vi "Open_File_for_write_check.vi"(8 "advisory dialog? (display:T)":bool=TRUE, 9 "append to file? (new file:F)":bool, 11 "file path":path) -> (0 "error out":errorcluster, 3 "refnum":refnum<file>)   [LabVIEW 2015]
doc: "Opens an existing file, creates a new file, or replaces an existing file, programmatically or interactively using dialog. You can optionally specify a dialog prompt, default file name, start path, or filter pattern, and you can specify open and deny modes when opening a file, plus group and permission when creating a new file. Use this VI with the intermediate Write File+ or Read File+ VIs described below.\n\nfile path is the path name of the file. If file path is empty (default value) or is Not A Path, the VI displays a File dialog box from which you can select a file. Error 43 occurs if the user cancels the dialog. \n\nfunction is the operation to perform:\n\n 0 (open) opens an existing file. Error 7 occurs if the file cannot be found.\n \n 1 (open or create) opens an existing file or creates a new file if one does not exist.\n\n 2 (create or replace) creates a new file or replaces a file if it exists and you give permission. Replacement is done by opening the file and setting EOF to 0. Error 43 occurs if the user elects to disallow the replacement using dialog. \n\n 3 (create) creates a new file. Error 8 occurs if the file already exists.\n\nadvisory dialog? Set TRUE (default) if you want a dialog if function=0 and the file does not exist, or if function=2 or 3 and the file exists.\n\nprompt is the message that appears below the list of files and directories in the file dialog.\n\ndefault name is the initial file name that appears in the selection box of the file dialog.\n\nstart path is the path name to the initially displayed directory in a file dialog. The default value is Not A Path, which is the path to the last directory shown in a file dialog.\n\npattern is the match pattern specification to display only certain types of files or directories. See the description of the File Dialog function for more information.\n\nerror in is a cluster of three elements (error?, code, and source) that describe the upstream error state, that is, the existance of any error preceeding the execution of the VI. The VI executes normally only if no incoming error exists; otherwise it merely passes the error in value to error out. error? is TRUE if an error occurred; the default value is FALSE. code is the error code; the default value is 0. source is in most cases the name of the VI or function that produced the error; the default value is an empty string.\n\nnew file path is the path of the file opened or created. You can use this output to determine the path of a file that you open or create using dialog. new file path returns Not A Path if the user selects Cancel from the dialog box.\n\nrefnum is the reference number of the open file. The value is Not A Refnum if the file cannot be opened.\n\nfile size is the size of the file in bytes; it is also the location of the end of file.\n\nerror out is a cluster of three elements (error?, code, and source) that describe the error state following the execution of the VI. If an incoming error does not exist, the VI executes normally and error out describes the VI's error state; if an incoming error exists, error out equals error in."
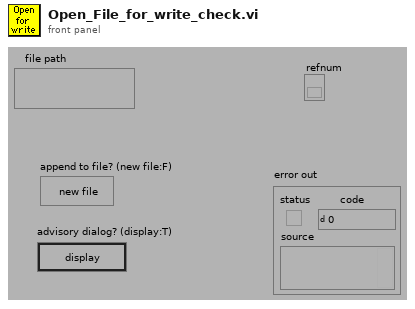
[diagram p1: front panel]
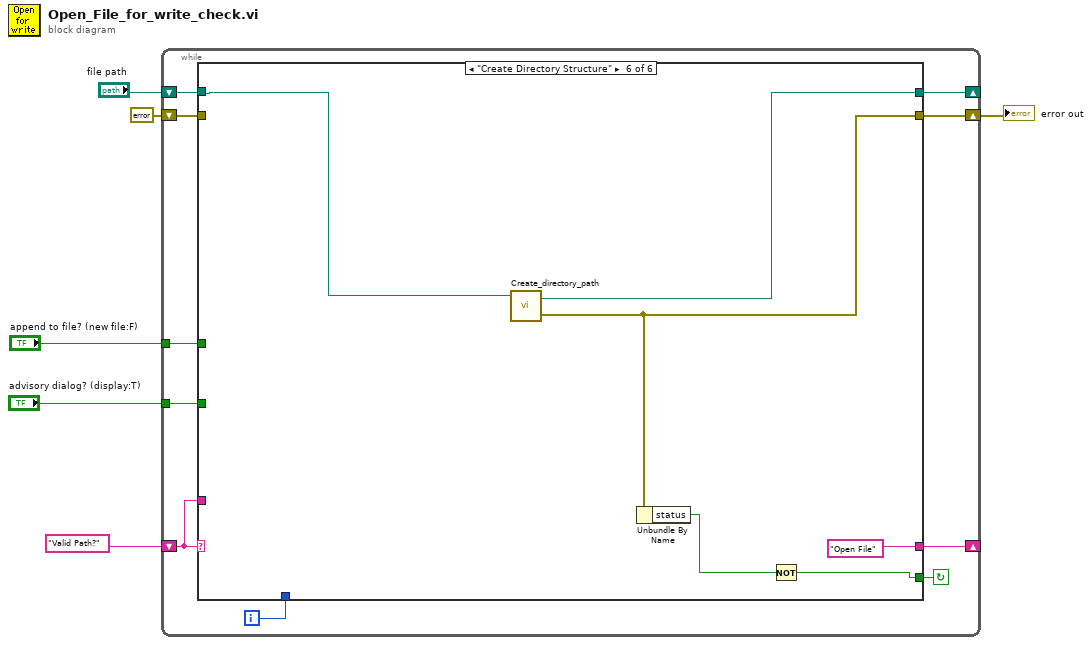
[diagram p0: block diagram]
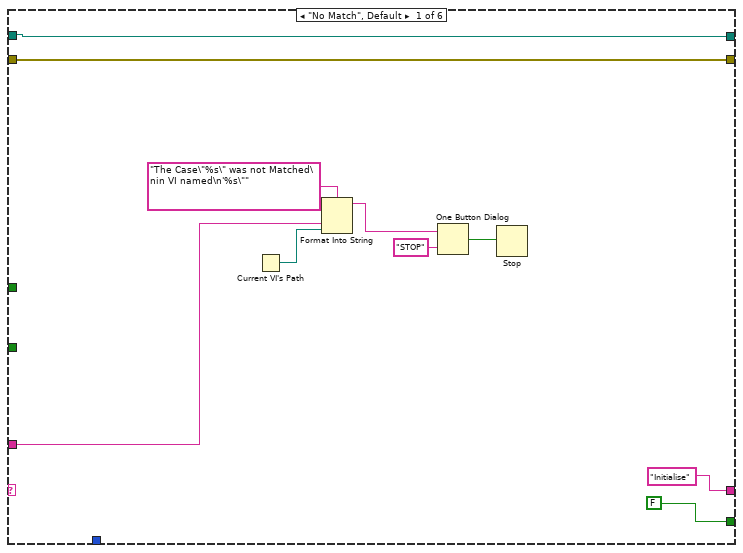
[diagram p2: hidden frame]
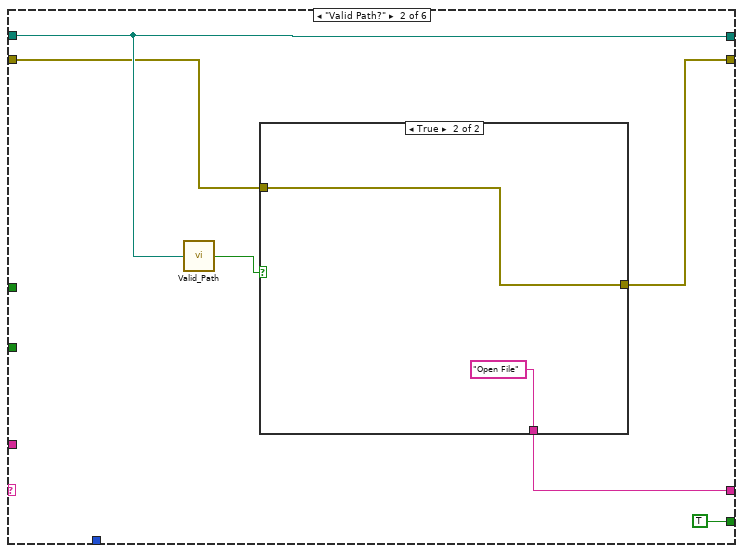
[diagram p3: hidden frame]
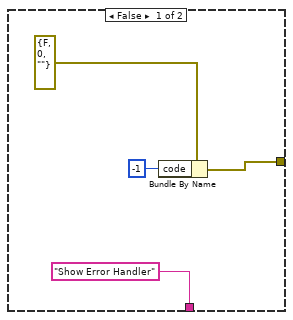
[diagram p4: hidden frame]
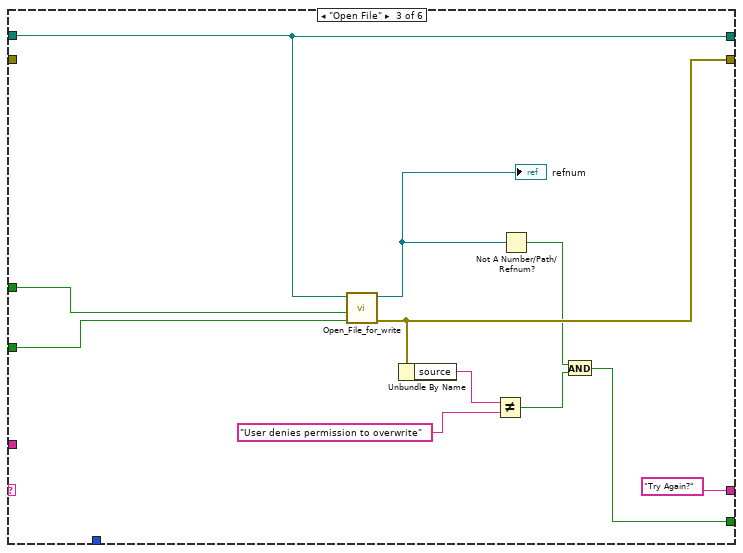
[diagram p5: hidden frame]
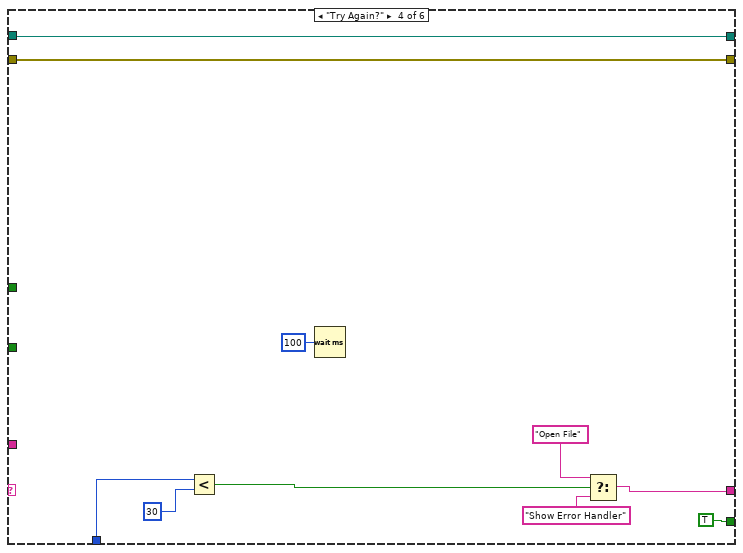
[diagram p6: hidden frame]
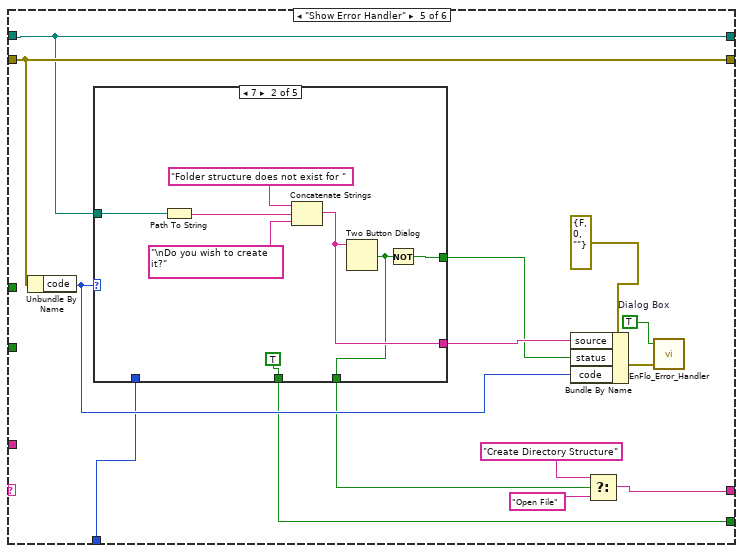
[diagram p7: hidden frame]
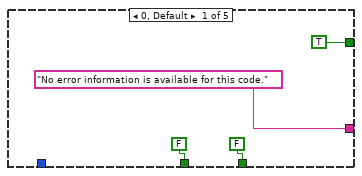
[diagram p8: hidden frame]
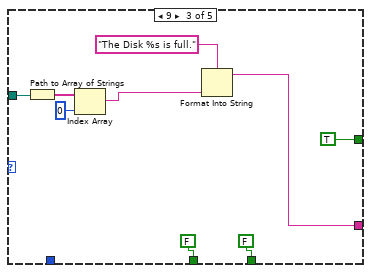
[diagram p9: hidden frame]
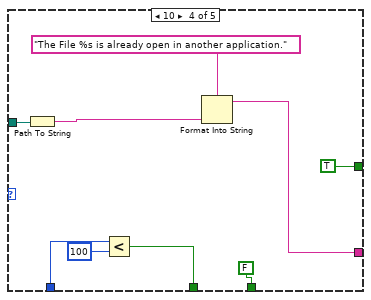
[diagram p10: hidden frame]
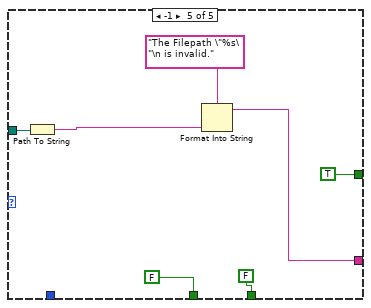
[diagram p11: hidden frame]
diagram:
  n1 = while {
    shift-left: "Valid Path?" -> [w14]
    shift-right: [w15] -> _
    tunnel: "append to file? (new file:F)" -> [w13]
    tunnel: "advisory dialog? (display:T)" -> [w12]
    shift-right: [w10] -> w3
    shift-left: errorcluster {"status"=FALSE, "code"=0, "source"=""} ("error out") -> [w7]
    shift-right: [w8] -> _
    shift-left: "file path" -> [w9]
    i -> [w11]
    stop <- w16 continue-if-true
    n2 = case shown="\"Create Directory Structure\"" w14 {
      tunnel: [FALSE TRUE w39 TRUE w61 w113] -> w16
      tunnel: ["Initialise" w30 "Try Again?" w54 w73 "Open File"] -> w15
      tunnel: w14 -> [w21 _ _ _ _ _]
      tunnel: w13 -> [_ _ w48 _ _ _]
      tunnel: w12 -> [_ _ w47 _ _ _]
      tunnel: w9 -> [w18 w32 w45 w50 w69 w115]
      tunnel: w11 -> [_ _ _ w57 w60 _]
      tunnel: [w17 w28 w44 w51 w70 w111] -> w10
      tunnel: [w18 w32 w45 w50 w69 w116] -> w8
      tunnel: w7 -> [w17 w27 _ w51 w70 _]
      frame "No Match", Default {
        n3 = Current VI's Path() -> (path=w20:path)
        n4 = Format Into String(format string="The Case\"%s\" was not Matched\nin VI named\n'%s\"" ("Format String"), w21, w20) -> (resulting string=w24:string)  [unwired: 2 in, 1 out]
        n5 = One Button Dialog(message=w24, button name ("OK")="STOP") -> (true=w22:bool)
        n6 = Stop(stop? (T)=w22) -> ()
      }
      frame "Valid Path?" {
        n7 = call "Valid_Path.vi"("Filename"=w32) -> ("Valid Path?"=w31:bool)
        n8 = case shown="True" w31 {
          tunnel: ["Show Error Handler" "Open File"] -> w30
          tunnel: [w35 w37] -> w28
          tunnel: w27 -> [_ w37]
          frame False {
            n9 = Bundle By Name(cluster=errorcluster {"status"=FALSE, "code"=0, "source"=""} ("error in (no error)"), "code"=-1) -> (w35:errorcluster)
          }
          frame True {
          }
        }
      }
      frame "Open File" {
        n10 = call "Open_File_for_write.vi"("advisory dialog? (display:T)"=w47, "append to file? (new file:F)"=w48, "file path"=w45) -> ("error out"=w44:errorcluster, "refnum"=w46:refnum<file>)  [unwired: 7 out]
        "refnum" <- w46
        n11 = Unbundle By Name(w44) -> ("source"=w42:string)
        n12 = Not Equal?(x=w42, y="User denies permission to overwrite") -> (x != y?=w41:bool)
        n13 = Not A Number/Path/Refnum?(number/path/refnum=w46) -> (NaN/Path/Refnum?=w40:bool)
        n14 = And(x=w40, y=w41) -> (x .and. y?=w39:bool)
      }
      frame "Try Again?" {
        n15 = Less?(x=w57, y=30) -> (x < y?=w55:bool)
        n16 = Wait (ms)(milliseconds to wait=u32 100) -> ()  [unwired: 1 out]
        n17 = Select(t="Open File", s=w55, f="Show Error Handler") -> (s? t:f=w54:string)
      }
      frame "Show Error Handler" {
        w68 = TRUE  # Dialog Box
        n18 = Unbundle By Name(w70) -> ("code"=w64:i32)
        n19 = case shown="7" w64 {
          tunnel: w69 -> [_ w82 w94 w103 w110]
          tunnel: ["No error information is available for this code." w81 w89 w101 w108] -> w65
          tunnel: [FALSE w79 FALSE FALSE FALSE] -> w63
          tunnel: [TRUE w80 TRUE TRUE TRUE] -> w62
          tunnel: [FALSE TRUE FALSE w95 FALSE] -> w61
          tunnel: w60 -> [_ _ _ w97 _]
          frame 0, Default {
          }
          frame 7 {
            n20 = Path To String(path=w82) -> (string=w84:string)
            n21 = Concatenate Strings("Folder structure does not exist for ", w84, "\nDo you wish to create it?") -> (w81:string)
            n22 = Two Button Dialog(message=w81) -> (T button?=w79:bool)  [unwired: 2 out]
            n23 = Not(x=w79) -> (.not. x?=w80:bool)
          }
          frame 9 {
            n24 = Path to Array of Strings(0:w94) -> (2:w93:string[])  [unwired: 1 out]
            n25 = Index Array(array=w93, index=0 ("Index")) -> (element=w91:string)
            n26 = Format Into String(format string="The Disk %s is full." ("Format String"), w91) -> (resulting string=w89:string)  [unwired: 2 in, 1 out]
          }
          frame 10 {
            n27 = Path To String(path=w103) -> (string=w100:string)
            n28 = Less?(x=w97, y=100) -> (x < y?=w95:bool)
            n29 = Format Into String(format string="The File %s is already open in another application." ("Format String"), w100) -> (resulting string=w101:string)  [unwired: 2 in, 1 out]
          }
          frame -1 {
            n30 = Path To String(path=w110) -> (string=w107:string)
            n31 = Format Into String(format string="The Filepath \"%s\"\n is invalid." ("Format String"), w107) -> (resulting string=w108:string)  [unwired: 2 in, 1 out]
          }
        }
        n32 = Bundle By Name(cluster=errorcluster {"status"=FALSE, "code"=0, "source"=""} ("error in (no error)"), "source"=w65, "status"=w62, "code"=w64) -> (w67:errorcluster)
        n33 = Select(t="Create Directory Structure", s=w63, f="Open File") -> (s? t:f=w73:string)
        n34 = call "EnFlo_Error_Handler.vi"("error in (no error)"=w67, "Dialog Box (T)"=w68) -> ()  [unwired: 1 in, 3 out]
      }
      frame "Create Directory Structure" {
        n35 = call "Create_directory_path.vi"("Path name"=w115) -> ("error out"=w111:errorcluster, "Path name Out"=w116:path)  [unwired: 2 in]
        n36 = Unbundle By Name(w111) -> ("status"=w112:bool)
        n37 = Not(x=w112) -> (.not. x?=w113:bool)
      }
    }
  }
  "error out" <- w3
